vi "Split Lines.vi"(11 "String":string) -> (3 "Array":string[](array[string]))   [LabVIEW 2017]
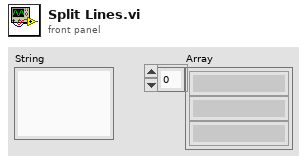
[diagram p1: front panel]
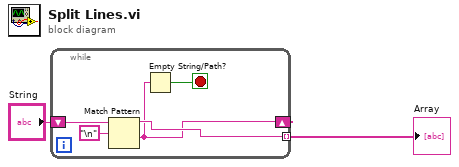
[diagram p0: block diagram]
diagram:
  n1 = while {
    tunnel: [w5] -> w2 mode=indexing
    shift-right: [w3] -> _
    shift-left: "String" -> [w7]
    stop <- w4 stop-if-true
    n2 = Match Pattern(string=w7, regular expression="\n") -> (before substring=w5:string, after substring=w3:string)  [unwired: 1 in, 2 out]
    n3 = Empty String/Path?(string/path=w3) -> (empty?=w4:bool)
  }
  "Array" <- w2
